vi "Load Bom into Array.vi"(0 "BOM":path) -> (1 "Text BOM":string[](array[string]), 2 "Cluster Bom":T1[](array[typedef]))   [LabVIEW 2013]
uses:
  BOM Item.ctl
  Controls/Components.ctl
  Controls/Component Sub Type.ctl
  <vilib>/Utility/file.llb/Read From Spreadsheet File (string).vi
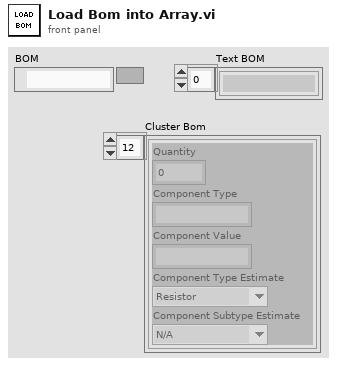
[diagram p1: front panel]
types:
  T1 = typedef "BOM Item.ctl" = cluster{"Quantity":i32, "Component Type":string, "Component Value":string, "Component Type Estimate":T2, "Component Subtype Estimate":T3}
  T2 = typedef "Components.ctl" = enum16{"Resistor", "Capacitor", "Diode", "Voltage Regulator", "Transistors", "ICs", "Misc"}
  T3 = typedef "Component Sub Type.ctl" = enum16{"N/A", "Carbon", "Variable - Trimmer", "Variable - Pot", "Ceramic", "Electrolitic", "Zenner", "TO-92", "TO-220", "NPN", "PNP", "CMOS", "Processor"}
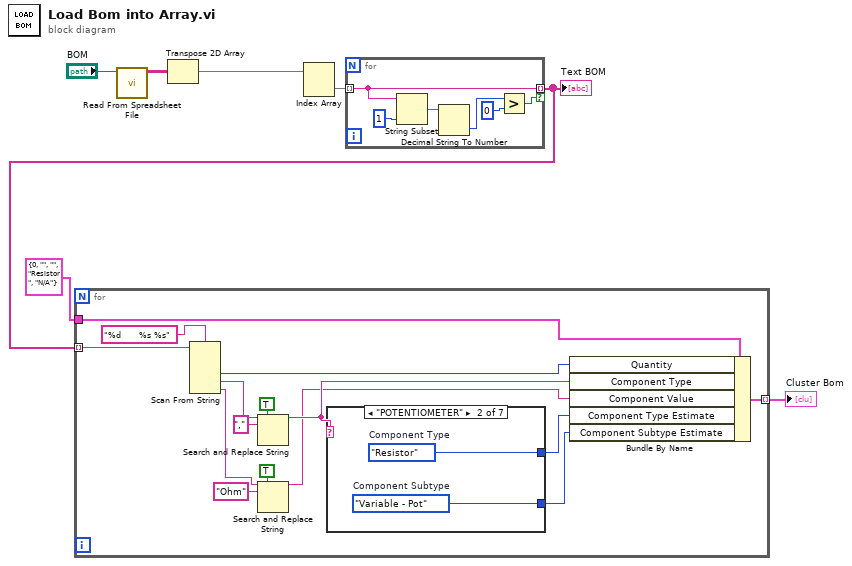
[diagram p0: block diagram]
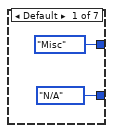
[diagram p2: hidden frame]
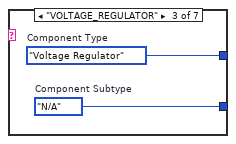
[diagram p3: hidden frame]
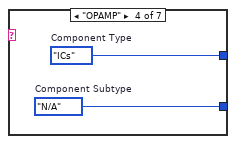
[diagram p4: hidden frame]
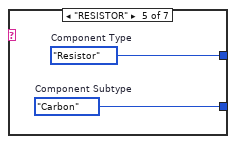
[diagram p5: hidden frame]
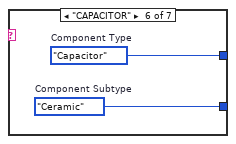
[diagram p6: hidden frame]
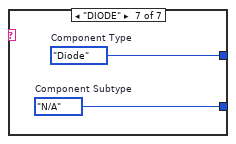
[diagram p7: hidden frame]
diagram:
  n1 = call-poly <vilib>:"Read From Spreadsheet File.vi"("file path (dialog if empty)"="BOM") -> ("all rows"=w5:string[][])  [unwired: 6 in, 4 out]
  n2 = Transpose 2D Array(2D array=w5) -> (transposed array=w6:string[][])
  n3 = Index Array(array=w6) -> (element=w7:string[])  [unwired: 2 in]
  n4 = for {
    tunnel: w7 -> [w9] mode=indexing
    tunnel: [w9] -> w1 mode=indexing if=w8
    n5 = String Subset(string=w9, length (rest)=1 ("length (rest)")) -> (substring=w12:string)  [unwired: 1 in]
    n6 = Decimal String To Number(string=w12) -> (number=w11:i32)  [unwired: 2 in, 1 out]
    n7 = Greater?(x=w11, y=0) -> (0:w8:bool)
  }
  "Text BOM" <- w1
  n8 = for {
    tunnel: w1 -> [w28] mode=indexing
    tunnel: T1 {"Quantity"=0, "Component Type"="", "Component Value"="", "Component Type Estimate"=enum."Resistor", "Component Subtype Estimate"=enum."N/A"} ("Cluster") -> [w26]
    tunnel: [w22] -> w2 mode=indexing
    n9 = Scan From String(format string="%d      %s %s", input string=w28) -> (output 1=w23:i32, output 2=w21:string, output 3=w15:string)  [unwired: 5 in, 3 out]
    n10 = Search and Replace String(replace all?=TRUE ("replace all? (F)"), input string=w21, search string=",") -> (result string=w18:string)  [unwired: 5 in, 3 out]
    n11 = Search and Replace String(replace all?=TRUE ("replace all? (F)"), input string=w15, search string="Ohm") -> (result string=w14:string)  [unwired: 5 in, 3 out]
    n12 = case shown="\"POTENTIOMETER\"" w18 {
      tunnel: [Components."Misc" ("Component Type") w32 w34 w36 w38 w40 w42] -> w25
      tunnel: [Component_Sub_Type."N/A" ("Component Subtype") w31 w33 w35 w37 w39 w41] -> w24
      frame Default {
      }
      frame "POTENTIOMETER" {
        w31 = Component_Sub_Type."Variable - Pot"  # Component Subtype
        w32 = Components."Resistor"  # Component Type
      }
      frame "VOLTAGE_REGULATOR" {
        w33 = Component_Sub_Type."N/A"  # Component Subtype
        w34 = Components."Voltage Regulator"  # Component Type
      }
      frame "OPAMP" {
        w35 = Component_Sub_Type."N/A"  # Component Subtype
        w36 = Components."ICs"  # Component Type
      }
      frame "RESISTOR" {
        w37 = Component_Sub_Type."Carbon"  # Component Subtype
        w38 = Components."Resistor"  # Component Type
      }
      frame "CAPACITOR" {
        w39 = Component_Sub_Type."Ceramic"  # Component Subtype
        w40 = Components."Capacitor"  # Component Type
      }
      frame "DIODE" {
        w41 = Component_Sub_Type."N/A"  # Component Subtype
        w42 = Components."Diode"  # Component Type
      }
    }
    n13 = Bundle By Name(cluster=w26, "Quantity"=w23, "Component Type"=w18, "Component Value"=w14, "Component Type Estimate"=w25, "Component Subtype Estimate"=w24) -> (w22:T1)
  }
  "Cluster Bom" <- w2
